vi "Defeated Message.vi"(11 "MyTeam in":refnum<class "MyTeam.lvclass">) -> (2 "Defeated Message":string)   [LabVIEW 2020, in "SquareTeam.lvlib" / "MyTeam.lvclass"]
uses:
  MyTeam.lvclass
  MyTeam.lvclass/MyTeam.ctl
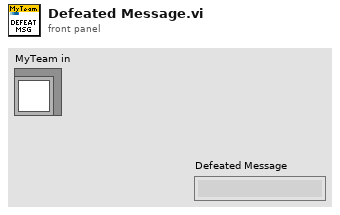
[diagram p1: front panel]
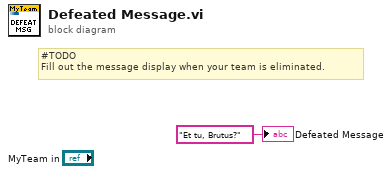
[diagram p0: block diagram]
diagram:
  # "#TODO\nFill out the message display when your team is eliminated."
  "Defeated Message" <- "Et tu, Brutus?" ("Defeated Message")
